vi "ClearOutputValuesOfDevices.vi"(11 "OutputValuesOfDevices":refnum<vi>) -> ()   [LabVIEW 2013]
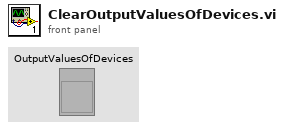
[diagram p1: front panel]
types:
  T1 = cluster{"KEITHLEY 2182 & KEITHLEY 6221":dbl[][], "Other Devices":dbl[][]}
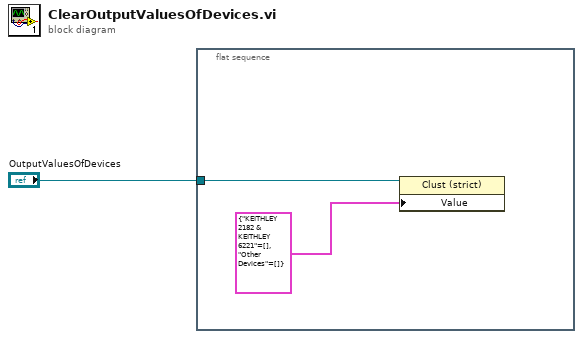
[diagram p0: block diagram]
diagram:
  n1 = flat-sequence {
    tunnel: "OutputValuesOfDevices" -> [w3]
    frame #0 {
      n2 = property class="Clust (strict)"(reference=w3, "Value"=T1 {"KEITHLEY 2182 & KEITHLEY 6221"=[], "Other Devices"=[]}) -> ()  [unwired: 1 in, 2 out]
    }
  }
